vi "DB Close.vi"(8 "error in (no error)":errorcluster, 11 "Db Reference":refnum<k24>) -> (0 "error out":errorcluster)   [LabVIEW 2020]
uses:
  D:/Labview/Auto Run Screen/Source Code/Database/Support/dbquery.dll
  Support/dbquery.dll
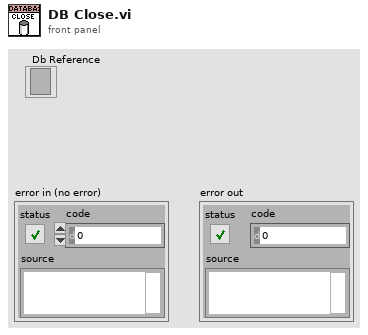
[diagram p1: front panel]
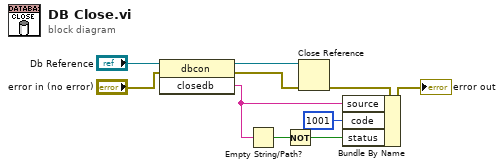
[diagram p0: block diagram]
diagram:
  n1 = invoke class="dbcon" method="closedb"(reference="Db Reference", error in="error in (no error)") -> (reference out=w8:refnum<k24>, error out=w6:errorcluster, "closedb"=w3:string)  [unwired: 1 in]
  n2 = Empty String/Path?(string/path=w3) -> (empty?=w2:bool)
  n3 = Not(x=w2) -> (.not. x?=w1:bool)
  n4 = Close Reference(reference=w8, error in (no error)=w6) -> (error out=w10:errorcluster)
  n5 = Bundle By Name(cluster=w10, "source"=w3, "code"=1001, "status"=w1) -> (→"error out":errorcluster)
